vi "Start JAUS Test.vi"() -> ()   [LabVIEW 2009]
uses:
  <vilib>/Platform/TimedLoop/XDataNode/XDataNode.xnode
  <vilib>/Platform/TimedLoop/XDataNode/loadlvalarms.vi
  <vilib>/Platform/TimedLoop/XDataNode/timing_clust.ctl
  <vilib>/Platform/TimedLoop/XDataNode/nitl_modes.ctl
  <vilib>/Platform/TimedLoop/XDataNode/wakeup.ctl
  <vilib>/Platform/TimedLoop/XDataNode/XDNodeRunTimeDep.lvlib
panel:
  out "Array":T1(array[cluster])
  in  "Kill All":bool
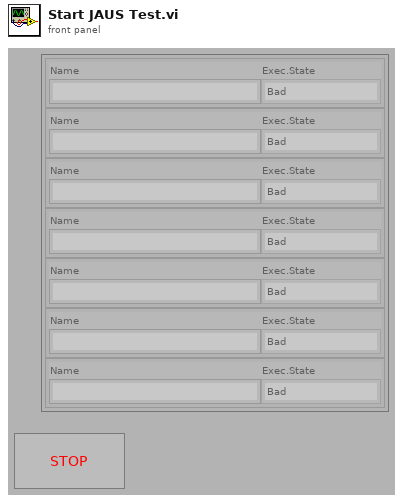
[diagram p1: front panel]
types:
  T1 = cluster{"Name":string, "Exec.State":enum32{"Bad", "Idle", "Run top level", "Running"}}[]
  T2 = typedef "XDNodeRunTimeDep.lvlib/timing_clust.ctl" = cluster{"Expected End [f-1]":u64, "Actual End [f-1]":u64, "Finished Late? [f-1]":bool, "Expected End [i-1]":u64, "Actual End [i-1]":u64, "Finished Late? [i-1]":bool, "Expected Start [i]":u64, "Actual Start [i]":u64, "Expected Start [f]":u64, "Actual Start [f]":u64, "Source Name":string, "Structure Name":string, "Period":i64, "Deadline":i64, "Offset":i64, "Start":i64, "Priority":i32, "Timeout":i32, "Mode":T3, "Wakeup Reason":T4, "Error":errorcluster, "Source Type":string, "Secondary Source Type":string, "Global End Time":u64, "Global Start Time":u64, "Frame Duration":u64, "Iteration Duration":u64, "Assigned CPU":i32, "I/O Scan Engine Mode":u32}
  T3 = typedef "XDNodeRunTimeDep.lvlib/nitl_modes.ctl" = enum32{"No Change", "Process missed periods, maintain original phase", "Discard missed periods, maintain original phase", "Process missed periods, ignore original phase", "Discard missed periods, ignore original phase"}
  T4 = typedef "XDNodeRunTimeDep.lvlib/wakeup.ctl" = enum32{"Normal", "Aborted", "Asynchronous wakeup", "Timing source error", "Timed loop error", "Timeout"}
  T5 = enum32{"Bad", "Idle", "Run top level", "Running"}
  T6 = cluster{"Name":string, "Exec.State":enum32{"Bad", "Idle", "Run top level", "Running"}}
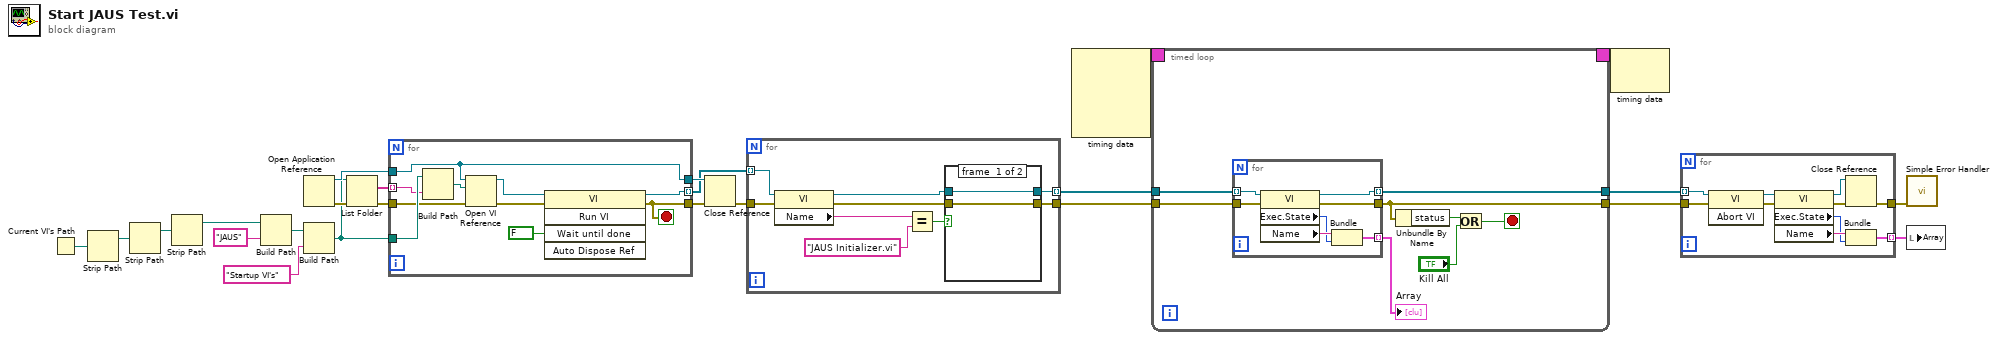
[diagram p0: block diagram]
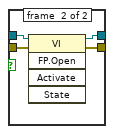
[diagram p2: hidden frame]
diagram:
  n1 = Current VI's Path() -> (path=w6:path)
  n2 = Strip Path(path=w6) -> (stripped path=w24:path)  [unwired: 1 out]
  n3 = Strip Path(path=w24) -> (stripped path=w13:path)  [unwired: 1 out]
  n4 = Strip Path(path=w13) -> (stripped path=w12:path)  [unwired: 1 out]
  n5 = Build Path(base path=w12, name or relative path="JAUS") -> (appended path=w9:path)
  n6 = Open Application Reference() -> (0:w21:errorcluster, 3:w23:refnum<vi>)  [unwired: 4 in]
  n7 = Build Path(base path=w9, name or relative path="Startup VI's") -> (appended path=w8:path)
  n8 = List Folder(path=w8, error in=w21) -> (filenames=w22:string[], error out=w20:errorcluster)  [unwired: 2 in, 2 out]
  n9 = for {
    tunnel: w23 -> [w25]
    tunnel: w8 -> [w34]
    tunnel: w22 -> [w33] mode=indexing
    tunnel: w20 -> [w31]
    tunnel: [w29] -> w4 mode=indexing
    tunnel: [w26] -> w7
    tunnel: [w25] -> w11
    stop <- w26 stop-if-true
    n10 = Build Path(base path=w34, name or relative path=w33) -> (appended path=w32:path)
    n11 = Open VI Reference(application reference (local)=w25, vi path=w32, error in (no error)=w31) -> (vi reference=w30:refnum<vi>, error out=w28:errorcluster)  [unwired: 3 in]
    n12 = invoke class="VI" method="Run VI"(reference=w30, error in=w28, "Wait until done"=FALSE ("Wait Until Done")) -> (reference out=w29:refnum<vi>, error out=w26:errorcluster)  [unwired: 2 in, 3 out]
  }
  n13 = Close Reference(reference=w11, error in (no error)=w7) -> (error out=w1:errorcluster)
  n14 = for {
    tunnel: w4 -> [w43] mode=indexing
    tunnel: w1 -> [w42]
    tunnel: [w37] -> w2
    tunnel: [w36] -> w3 mode=indexing
    n15 = property class="VI"(reference=w43, error in=w42) -> (reference out=w39:refnum<vi>, error out=w38:errorcluster, "Name"=w41:string)
    n16 = Equal?(x=w41, y="JAUS Initializer.vi") -> (x = y?=w35:bool)
    n17 = case shown="False" w35 {
      tunnel: w39 -> [w45 w49]
      tunnel: w38 -> [w44 w48]
      tunnel: [w44 w47] -> w37
      tunnel: [w45 w46] -> w36
      frame #0 {
      }
      frame #1 {
        n18 = invoke class="VI" method="FP.Open"(reference=w49, error in=w48) -> (reference out=w46:refnum<vi>, error out=w47:errorcluster)  [unwired: 3 in, 3 out]
      }
    }
  }
  n19 = node-c288() -> (w16:T2)  [unwired: 4 in]
  n20 = timed-loop {
    tunnel: w3 -> [w56]
    tunnel: [w54] -> w19
    tunnel: w2 -> [w55]
    tunnel: [w51] -> w18
    timing: w16 -> [_]
    timing-out: [_] -> w15
    stop <- w53 stop-if-true
    n21 = for {
      tunnel: w56 -> [w64] mode=indexing
      tunnel: w55 -> [w63]
      tunnel: [w62] -> w51
      tunnel: [w61] -> w54 mode=indexing
      tunnel: [w58] -> w50 mode=indexing
      n22 = property class="VI"(reference=w64, error in=w63) -> (reference out=w61:refnum<vi>, error out=w62:errorcluster, "Exec.State"=w59:T5, "Name"=w60:string)
      n23 = Bundle("Name"=w60, "Exec.State"=w59) -> (w58:T6)  [unwired: 1 in]
    }
    "Array" <- w50
    n24 = Unbundle By Name(w51) -> ("status"=w52:bool)
    n25 = Or(x=w52, y="Kill All") -> (x .or. y?=w53:bool)
  }
  n26 = node-c288(w15) -> ()  [unwired: 1 out]
  n27 = for {
    tunnel: w19 -> [w76] mode=indexing
    tunnel: w18 -> [w75]
    tunnel: [w74] -> w17
    tunnel: [w67] -> w5 mode=indexing
    n28 = invoke class="VI" method="Abort VI"(reference=w76, error in=w75) -> (reference out=w71:refnum<vi>, error out=w70:errorcluster)  [unwired: 1 in, 1 out]
    n29 = property class="VI"(reference=w71, error in=w70) -> (reference out=w69:refnum<vi>, error out=w68:errorcluster, "Exec.State"=w72:T5, "Name"=w73:string)
    n30 = Close Reference(reference=w69, error in (no error)=w68) -> (error out=w74:errorcluster)
    n31 = Bundle("Name"=w73, "Exec.State"=w72) -> (w67:T6)  [unwired: 1 in]
  }
  n32 = call <vilib>:"Simple Error Handler.vi"("error in (no error)"=w17) -> ()  [unwired: 4 in, 5 out]
  n33 = local write "Array"(w5) -> ()
